vi "Get All Outgoing Frames.vi"(8 "error in":errorcluster, 11 "Item Ref":T3 format="%.0x") -> (0 "error out":errorcluster, 2 "Frames":T2(array[cluster]), 3 "Item Ref out":T3 format="%.0x")   [LabVIEW 2019, in "J1939 Addon System Explorer.lvlib"]
uses:
  J1939 Addon System Explorer.lvlib
  <vilib>/NI VeriStand/Custom Device API/Custom Device Item Ref.ctl
  Addon Shared/Types/SPN Properties.ctl
  Addon Shared/SubVIs/Constants.vi
  <vilib>/NI VeriStand/Custom Device Tools/Custom Device Utility Library/NI VeriStand - Search for All Items by GUID.vi
  <vilib>/NI VeriStand/Custom Device API/Get Item Property (U32).vi
  <vilib>/NI VeriStand/Custom Device API/Get Item Property (Variant).vi
  Addon Shared/J1939 Addon Shared.lvlib
  <vilib>/NI VeriStand/Custom Device Tools/Custom Device Utility Library/Custom Device Utility Library.lvlib
  <vilib>/NI VeriStand/Custom Device API/Custom Device API.lvlib
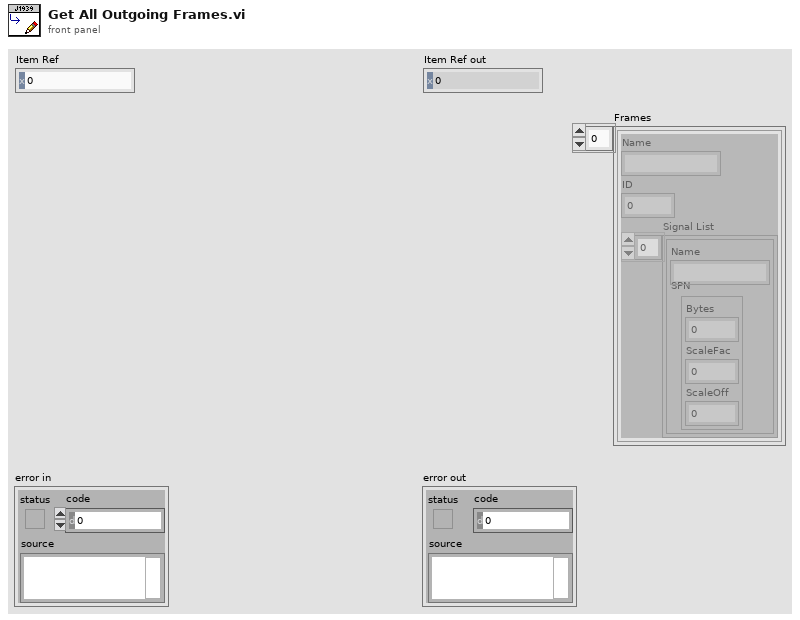
[diagram p1: front panel]
types:
  T1 = typedef "J1939 Addon Shared.lvlib/SPN Properties.ctl" = cluster{"Bytes":u32, "ScaleFac":dbl, "ScaleOff":dbl}
  T2 = cluster{"Name":string, "ID":u32, "Signal List":cluster{"Name":string, "SPN":T1}[]}[]
  T3 = typedef "Custom Device API.lvlib/Custom Device Item Ref.ctl" = u64
  T4 = typedef "Custom Device API.lvlib/Custom Device Item Info.ctl" = cluster{"Name":string, "Is Channel":bool, "GUID":string, "Is Waveform":bool}
  T5 = cluster{"Name":string, "Value":u32, cluster{"Name":string, "cluster":T1}[]}
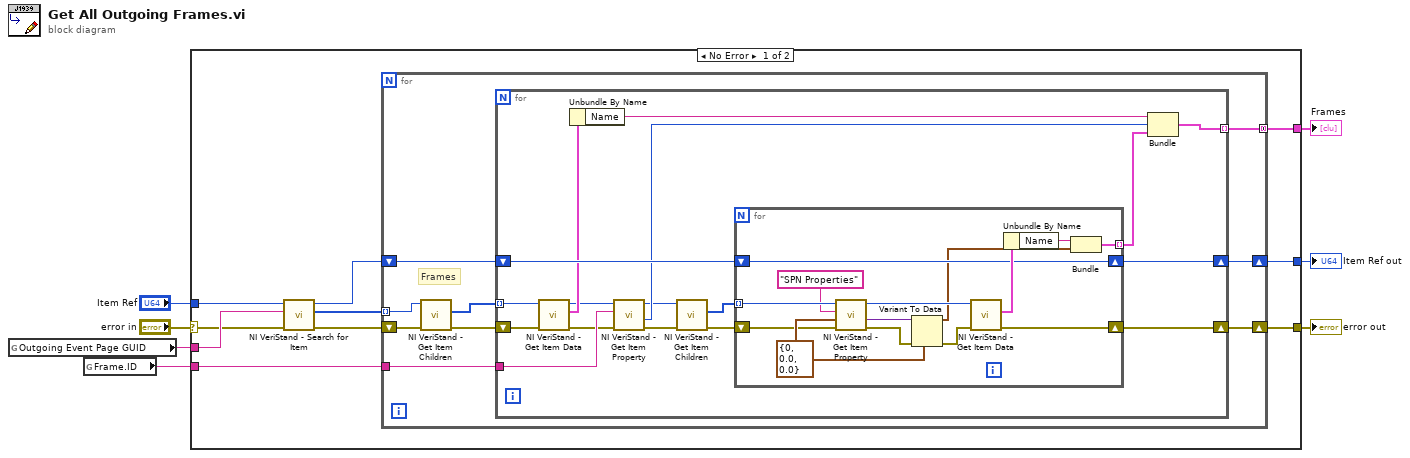
[diagram p0: block diagram]
diagram:
  n1 = global read "Constants.vi" "Outgoing Event Page GUID"() -> (w3:string)
  n2 = global read "Constants.vi" "Frame.ID"() -> (w6:string)
  n3 = case shown="No Error" "error in" {
    selector: "error in" -> [w12 w59]
    tunnel: [w9 w58] -> w7
    tunnel: w6 -> [w17 _]
    tunnel: [w10 w59] -> w5
    tunnel: "Item Ref" -> [w11 w58]
    tunnel: w3 -> [w16 _]
    tunnel: [w8 _] -> w1
    frame No Error {
      n4 = call-poly <vilib>:"NI VeriStand - Search for Item.vi"("error in"=w12, "Item GUID"=w16, "Section Ref in"=w11) -> ("error out"=w15:errorcluster, "Item Refs"=w13:T3[], "Section Ref out"=w14:T3)  [unwired: 5 in, 1 out]
      n5 = for {
        tunnel: w17 -> [w26]
        tunnel: [w22] -> w8 mode=concatenating
        shift-right: [w21] -> w9
        shift-left: w14 -> [w19]
        shift-right: [w23] -> w10
        shift-left: w15 -> [w20]
        tunnel: w13 -> [w18] mode=indexing
        # "Frames"
        n6 = call <vilib>:"NI VeriStand - Get Item Children.vi"("error in (no error)"=w20, "Item Ref in"=w18) -> ("error out"=w24:errorcluster, "Child Refs"=w25:T3[])  [unwired: 6 in, 2 out]
        n7 = for {
          shift-right: [w33] -> w23
          shift-left: w24 -> [w37]
          tunnel: w25 -> [w38] mode=indexing
          tunnel: w26 -> [w43]
          shift-right: [w40] -> w21
          shift-left: w19 -> [w41]
          tunnel: [w30] -> w22 mode=indexing
          n8 = call <vilib>:"NI VeriStand - Get Item Data.vi"("error in (no error)"=w37, "Item Ref in"=w38) -> ("error out"=w34:errorcluster, "Item Info"=w36:T4, "Item Ref out"=w35:T3)  [unwired: 6 in, 1 out]
          n9 = Unbundle By Name(w36) -> ("Name"=w32:string)
          n10 = call-poly <vilib>:"NI VeriStand - Get Item Property.vi"("error in (no error)"=w34, "Property Name"=w43, "Item Ref in"=w35) -> ("error out"=w28:errorcluster, "Value"=w31:u32, "Item Ref out"=w27:T3)  [unwired: 5 in, 1 out]
          n11 = call <vilib>:"NI VeriStand - Get Item Children.vi"("error in (no error)"=w28, "Item Ref in"=w27) -> ("error out"=w42:errorcluster, "Child Refs"=w39:T3[])  [unwired: 6 in, 2 out]
          n12 = for {
            shift-right: [w55] -> w33
            shift-left: w42 -> [w51]
            tunnel: w39 -> [w50] mode=indexing
            shift-right: [w56] -> w40
            shift-left: w41 -> [w56]
            tunnel: [w45] -> w29 mode=indexing
            w52 = T1 {"Bytes"=0, "ScaleFac"=0.0, "ScaleOff"=0.0} ("cluster")
            n13 = call-poly <vilib>:"NI VeriStand - Get Item Property.vi"("error in (no error)"=w51, "Default Value"=w52, "Property Name"="SPN Properties" ("SPN Properties"), "Item Ref in"=w50) -> ("error out"=w53:errorcluster, "Value"=w54:variant, "Item Ref out"=w49:T3)  [unwired: 4 in, 1 out]
            n14 = Variant To Data(error in=w53, type=w52, Variant=w54) -> (data=w47:T1, error out=w48:errorcluster)
            n15 = call <vilib>:"NI VeriStand - Get Item Data.vi"("error in (no error)"=w48, "Item Ref in"=w49) -> ("error out"=w55:errorcluster, "Item Info"=w57:T4)  [unwired: 6 in, 2 out]
            n16 = Unbundle By Name(w57) -> ("Name"=w46:string)
            n17 = Bundle("Name"=w46, "cluster"=w47) -> (w45:cluster{"Name":string, "cluster":T1})  [unwired: 1 in]
          }
          n18 = Bundle("Name"=w32, "Value"=w31, w29) -> (w30:T5)  [unwired: 1 in]
        }
      }
    }
    frame Error {
    }
  }
  "error out" <- w5
  "Item Ref out" <- w7
  "Frames" <- w1
